vi "多功能信号发生器及示波器.vi"() -> ()   [LabVIEW 2018]
uses:
  <vilib>/measure/NI_MABase.lvlib
panel:
  out "发生器":waveform(dbl)[](graph) caption="波形图"
  in  "三角波颜色":u32(colorbox)
  in  "方波颜色":u32(colorbox)
  in  "三角波显示":bool
  in  "方波显示":bool
  in  "正弦波颜色":u32(colorbox)
  in  "正弦波显示":bool
  in  "时间上限":dbl=1000.0
  in  "幅值上限":dbl=1.0
  in  "幅值下限":dbl=-1.0
  in  "时间下限":dbl
  in  "波形选择":T1(ring)
  in  "幅值":dbl
  in  "频率":dbl
  in  "停止":bool
  out "示波器":waveform(dbl)[](graph) caption="波形图"
  # "多功能\n示波器"
  # "多功能\n信号发生器"
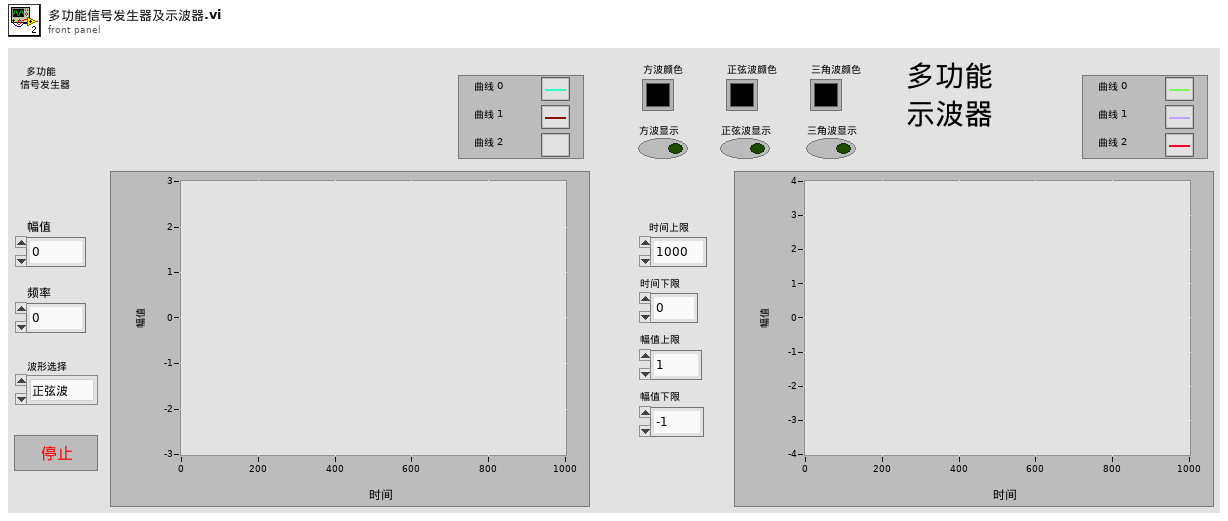
[diagram p1: front panel]
types:
  T1 = enum16{"正弦波", "三角波", "正三波", "方波", "方正波", "方三波", "三波形"}
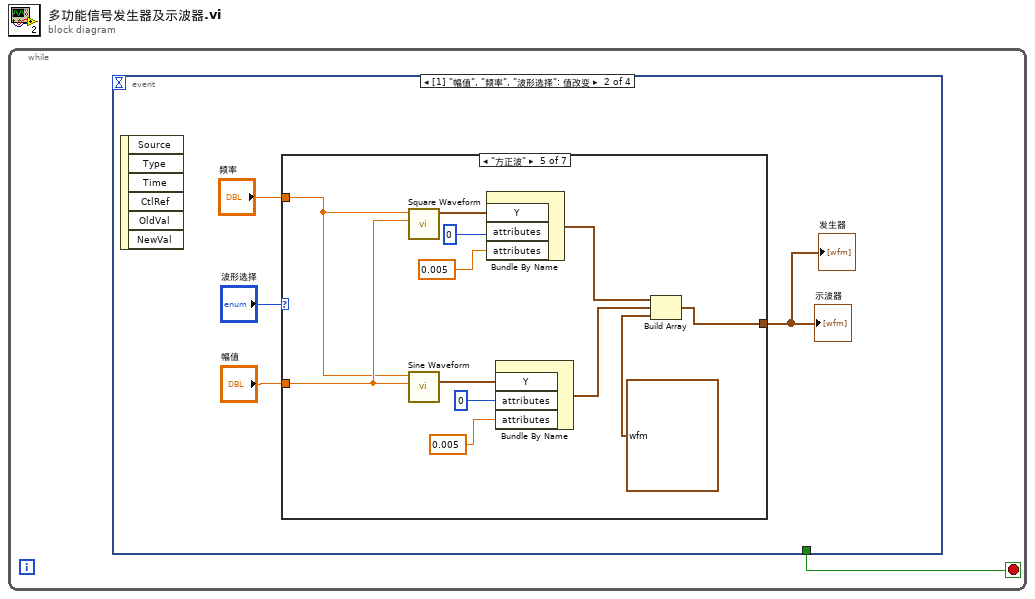
[diagram p0: block diagram]
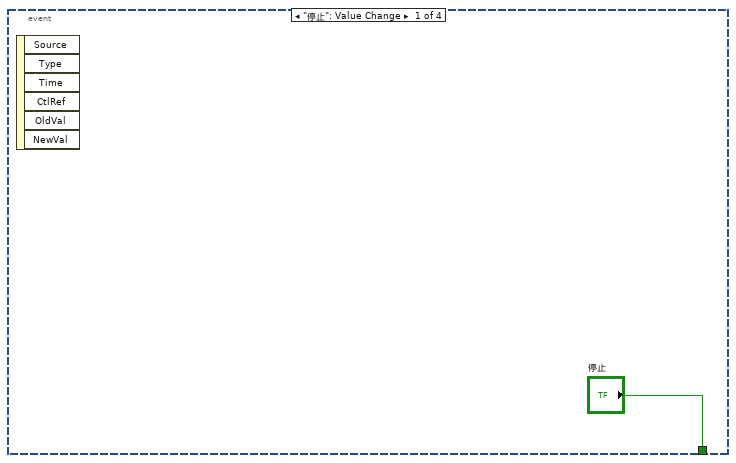
[diagram p2: hidden frame]
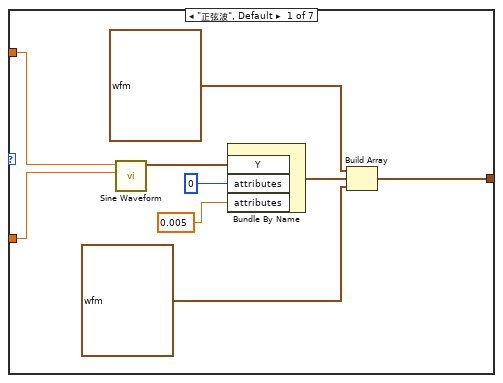
[diagram p3: hidden frame]
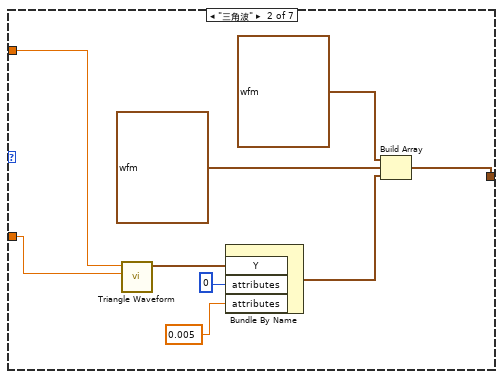
[diagram p4: hidden frame]
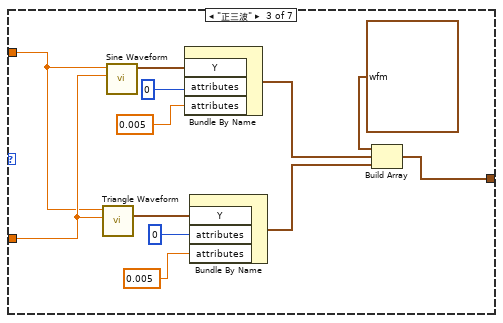
[diagram p5: hidden frame]
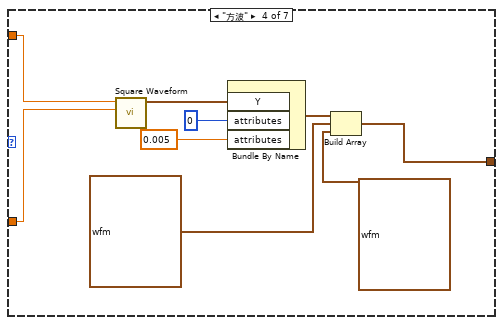
[diagram p6: hidden frame]
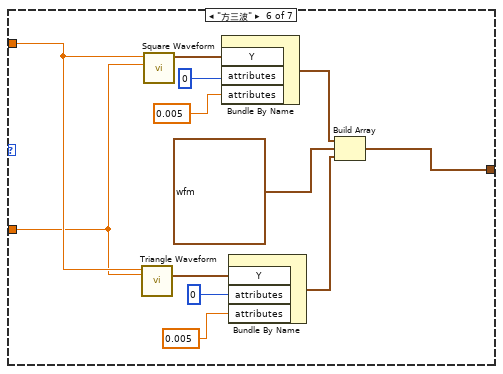
[diagram p7: hidden frame]
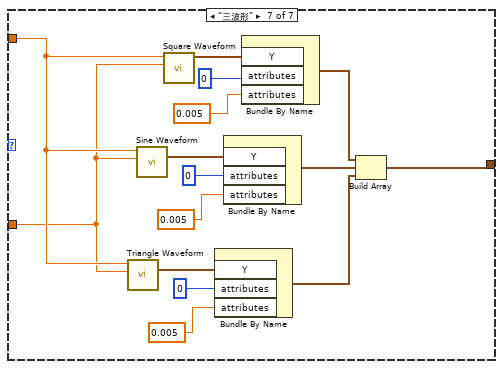
[diagram p8: hidden frame]
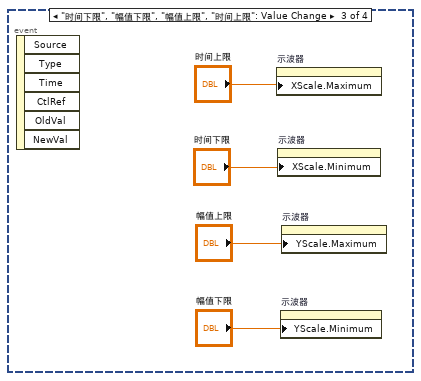
[diagram p9: hidden frame]
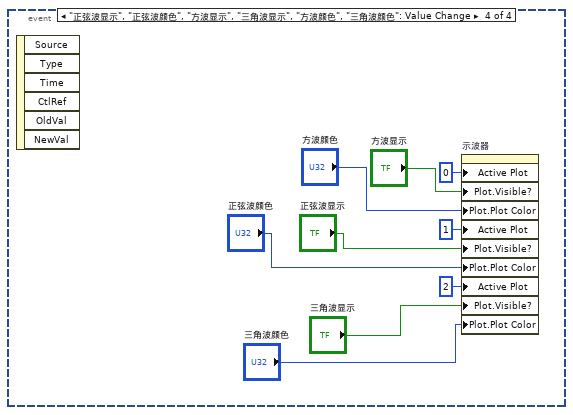
[diagram p10: hidden frame]
diagram:
  n1 = while {
    stop <- w1 stop-if-true
    n2 = event shown="[1] \"幅值\", \"频率\", \"波形选择\": 值改变" {
      selector: _ -> [_ _ _ _]
      dyn-events: _ -> [_ _ _ _]
      timeout: _ -> [_ _ _ _]
      tunnel: ["停止" _ _ _] -> w1
      event "停止": Value Change {
        n3 = event-data() -> ()  [unwired: 1 in, 6 out]
      }
      event "幅值", "频率", "波形选择": Value Change {
        n4 = event-data() -> ()  [unwired: 1 in, 6 out]
        n5 = case shown="\"方正波\"" "波形选择" {
          tunnel: "幅值" -> [w15 w20 w36 w40 w48 w60 w71]
          tunnel: "频率" -> [w14 w19 w35 w39 w47 w61 w72]
          tunnel: [w10 w18 w31 w41 w49 w62 w70] -> w3
          frame "正弦波", Default {
            n6 = call <vilib>:"Sine Waveform.vi"("amplitude"=w15, "frequency"=w14) -> ("signal out"=w11:waveform(dbl))  [unwired: 8 in, 1 out]
            n7 = Bundle By Name("Y"=w11, "attributes"=0, "attributes"=0.005) -> (w9:waveform(dbl))  [unwired: 1 in]
            n8 = Build Array(waveform(dbl) {"t0"=timestamp(0 s since 1904-01-01), "dt"=1.0, "Y"=[]} ("元素"), w9, waveform(dbl) {"t0"=timestamp(0 s since 1904-01-01), "dt"=1.0, "Y"=[]} ("元素")) -> (w10:waveform(dbl)[])
          }
          frame "三角波" {
            n9 = call <vilib>:"Triangle Waveform.vi"("amplitude"=w20, "frequency"=w19) -> ("signal out"=w22:waveform(dbl))  [unwired: 8 in, 1 out]
            n10 = Bundle By Name("Y"=w22, "attributes"=0, "attributes"=0.005) -> (w21:waveform(dbl))  [unwired: 1 in]
            n11 = Build Array(waveform(dbl) {"t0"=timestamp(0 s since 1904-01-01), "dt"=1.0, "Y"=[]} ("元素"), waveform(dbl) {"t0"=timestamp(0 s since 1904-01-01), "dt"=1.0, "Y"=[]} ("元素"), w21) -> (w18:waveform(dbl)[])
          }
          frame "正三波" {
            n12 = call <vilib>:"Triangle Waveform.vi"("amplitude"=w36, "frequency"=w35) -> ("signal out"=w28:waveform(dbl))  [unwired: 8 in, 1 out]
            n13 = call <vilib>:"Sine Waveform.vi"("amplitude"=w36, "frequency"=w35) -> ("signal out"=w34:waveform(dbl))  [unwired: 8 in, 1 out]
            n14 = Bundle By Name("Y"=w34, "attributes"=0, "attributes"=0.005) -> (w32:waveform(dbl))  [unwired: 1 in]
            n15 = Bundle By Name("Y"=w28, "attributes"=0, "attributes"=0.005) -> (w27:waveform(dbl))  [unwired: 1 in]
            n16 = Build Array(waveform(dbl) {"t0"=timestamp(0 s since 1904-01-01), "dt"=1.0, "Y"=[]} ("元素"), w32, w27) -> (w31:waveform(dbl)[])
          }
          frame "方波" {
            n17 = call <vilib>:"Square Waveform.vi"("amplitude"=w40, "frequency"=w39) -> ("signal out"=w43:waveform(dbl))  [unwired: 8 in, 1 out]
            n18 = Bundle By Name("Y"=w43, "attributes"=0, "attributes"=0.005) -> (w42:waveform(dbl))  [unwired: 1 in]
            n19 = Build Array(w42, waveform(dbl) {"t0"=timestamp(0 s since 1904-01-01), "dt"=1.0, "Y"=[]} ("元素"), waveform(dbl) {"t0"=timestamp(0 s since 1904-01-01), "dt"=1.0, "Y"=[]} ("元素")) -> (w41:waveform(dbl)[])
          }
          frame "方正波" {
            n20 = call <vilib>:"Square Waveform.vi"("amplitude"=w48, "frequency"=w47) -> ("signal out"=w57:waveform(dbl))  [unwired: 8 in, 1 out]
            n21 = call <vilib>:"Sine Waveform.vi"("amplitude"=w48, "frequency"=w47) -> ("signal out"=w52:waveform(dbl))  [unwired: 8 in, 1 out]
            n22 = Bundle By Name("Y"=w57, "attributes"=0, "attributes"=0.005) -> (w55:waveform(dbl))  [unwired: 1 in]
            n23 = Bundle By Name("Y"=w52, "attributes"=0, "attributes"=0.005) -> (w51:waveform(dbl))  [unwired: 1 in]
            n24 = Build Array(w55, w51, waveform(dbl) {"t0"=timestamp(0 s since 1904-01-01), "dt"=1.0, "Y"=[]} ("元素")) -> (w49:waveform(dbl)[])
          }
          frame "方三波" {
            n25 = call <vilib>:"Triangle Waveform.vi"("amplitude"=w60, "frequency"=w61) -> ("signal out"=w64:waveform(dbl))  [unwired: 8 in, 1 out]
            n26 = call <vilib>:"Square Waveform.vi"("amplitude"=w60, "frequency"=w61) -> ("signal out"=w69:waveform(dbl))  [unwired: 8 in, 1 out]
            n27 = Bundle By Name("Y"=w69, "attributes"=0, "attributes"=0.005) -> (w67:waveform(dbl))  [unwired: 1 in]
            n28 = Bundle By Name("Y"=w64, "attributes"=0, "attributes"=0.005) -> (w59:waveform(dbl))  [unwired: 1 in]
            n29 = Build Array(w67, waveform(dbl) {"t0"=timestamp(0 s since 1904-01-01), "dt"=1.0, "Y"=[]} ("元素"), w59) -> (w62:waveform(dbl)[])
          }
          frame "三波形" {
            n30 = call <vilib>:"Triangle Waveform.vi"("amplitude"=w71, "frequency"=w72) -> ("signal out"=w79:waveform(dbl))  [unwired: 8 in, 1 out]
            n31 = call <vilib>:"Sine Waveform.vi"("amplitude"=w71, "frequency"=w72) -> ("signal out"=w74:waveform(dbl))  [unwired: 8 in, 1 out]
            n32 = call <vilib>:"Square Waveform.vi"("amplitude"=w71, "frequency"=w72) -> ("signal out"=w84:waveform(dbl))  [unwired: 8 in, 1 out]
            n33 = Bundle By Name("Y"=w79, "attributes"=0, "attributes"=0.005) -> (w77:waveform(dbl))  [unwired: 1 in]
            n34 = Bundle By Name("Y"=w74, "attributes"=0, "attributes"=0.005) -> (w73:waveform(dbl))  [unwired: 1 in]
            n35 = Bundle By Name("Y"=w84, "attributes"=0, "attributes"=0.005) -> (w82:waveform(dbl))  [unwired: 1 in]
            n36 = Build Array(w82, w73, w77) -> (w70:waveform(dbl)[])
          }
        }
        "示波器" <- w3
        "发生器" <- w3
      }
      event "时间下限", "幅值下限", "幅值上限", "时间上限": Value Change {
        n37 = event-data() -> ()  [unwired: 1 in, 6 out]
        n38 = property on="示波器" class="WFGraph (严格)"("XScale.Maximum"="时间上限") -> ()  [unwired: 2 in, 2 out]
        n39 = property on="示波器" class="WFGraph (严格)"("XScale.Minimum"="时间下限") -> ()  [unwired: 2 in, 2 out]
        n40 = property on="示波器" class="WFGraph (严格)"("YScale.Minimum"="幅值下限") -> ()  [unwired: 2 in, 2 out]
        n41 = property on="示波器" class="WFGraph (严格)"("YScale.Maximum"="幅值上限") -> ()  [unwired: 2 in, 2 out]
      }
      event "正弦波显示", "正弦波颜色", "方波显示", "三角波显示", "方波颜色", "三角波颜色": Value Change {
        n42 = event-data() -> ()  [unwired: 1 in, 6 out]
        n43 = property on="示波器" class="WFGraph (严格)"("Active Plot"=u32 0 ("活动曲线"), "Plot.Visible?"="方波显示", "Plot.Plot Color"="方波颜色", "Active Plot"=u32 1 ("活动曲线"), "Plot.Visible?"="正弦波显示", "Plot.Plot Color"="正弦波颜色", "Active Plot"=u32 2 ("活动曲线"), "Plot.Visible?"="三角波显示", "Plot.Plot Color"="三角波颜色") -> ()  [unwired: 2 in, 2 out]
      }
    }
  }
